vi "Clousure.vi"(8 "error in":errorcluster, 11 "NYStyleCheesePizza":refnum<class "NYStyleCheesePizza.lvclass">) -> (0 "error out":errorcluster, 3 "NYStyleCheesePizza":refnum<class "NYStyleCheesePizza.lvclass">)   [LabVIEW 2020, in "FactoryMethod.lvlib" / "PizzaFactoryMethod.lvlib" / "NYStyleCheesePizza.lvclass"]
uses:
  NYStyleCheesePizza.lvclass
  Pizza/Pizza.lvclass
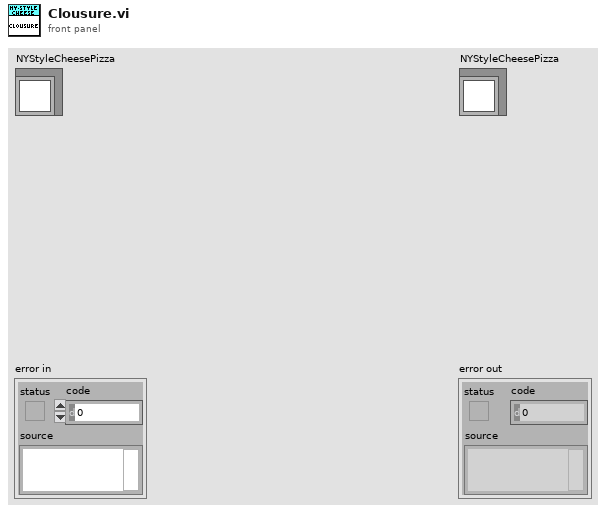
[diagram p1: front panel]
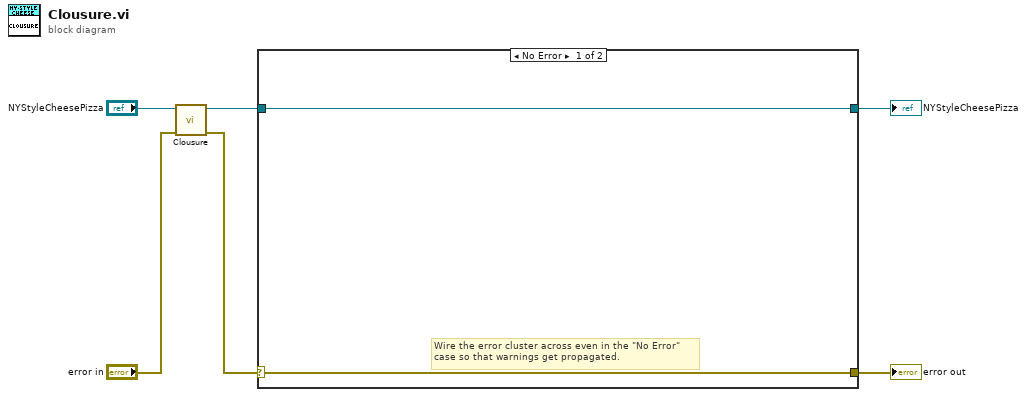
[diagram p0: block diagram]
diagram:
  n1 = call-parent "Clousure.vi"("error in (no error)"="error in", "Pizza"="NYStyleCheesePizza") -> ("error out"=w2:errorcluster, "Pizza"=w3:refnum<class "NYStyleCheesePizza.lvclass">)  [unwired: 8 in]
  n2 = case shown="No Error" w2 {
    selector: w2 -> [w7 w10]
    tunnel: [w7 w10] -> w5
    tunnel: [w8 w9] -> w6
    tunnel: w3 -> [w8 w9]
    frame No Error {
      # "Wire the error cluster across even in the \"No Error\"\ncase so that warnings get propagated."
    }
    frame Error {
    }
  }
  "error out" <- w5
  "NYStyleCheesePizza" <- w6
